vi "核查数据和日志信息出发送队列 (子VI).vi"() -> (0 "错误输出":errorcluster)   [LabVIEW 2016, in "数据传输系统.lvlib"]
uses:
  <vilib>/Utility/config.llb/NI_LVConfig.lvlib
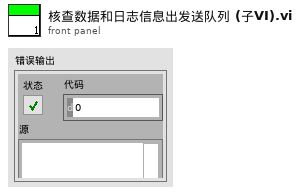
[diagram p1: front panel]
types:
  T1 = enum16{"质控数据", "操作日志", "仪器参数", "系统状态", "运行模式", "测量周期", "超标留样", "报警信息", "环境参数"}
  T2 = enum16{"空白测试", "跨度核查", "标样核查", "加标回收", "平行样", "集成干预"}
  T3 = typedef "NI_LVConfig.lvlib/Config Data RefNum.ctl" = refnum<k1>
  T4 = cluster{"PH":string[][], "CODCr":string[][], "氨氮":string[][], "CODMn":string[][], "总氮":string[][], "总磷":string[][], "电导率":string[][], "水温":string[][], "DO":string[][], "浊度":string[][], "叶绿素":string[][], "藻密度":string[][], "铜":string[][], "盐度":string[][], "水位":string[][], "流速":string[][], "瞬时流量":string[][], "累积流量":string[][]}
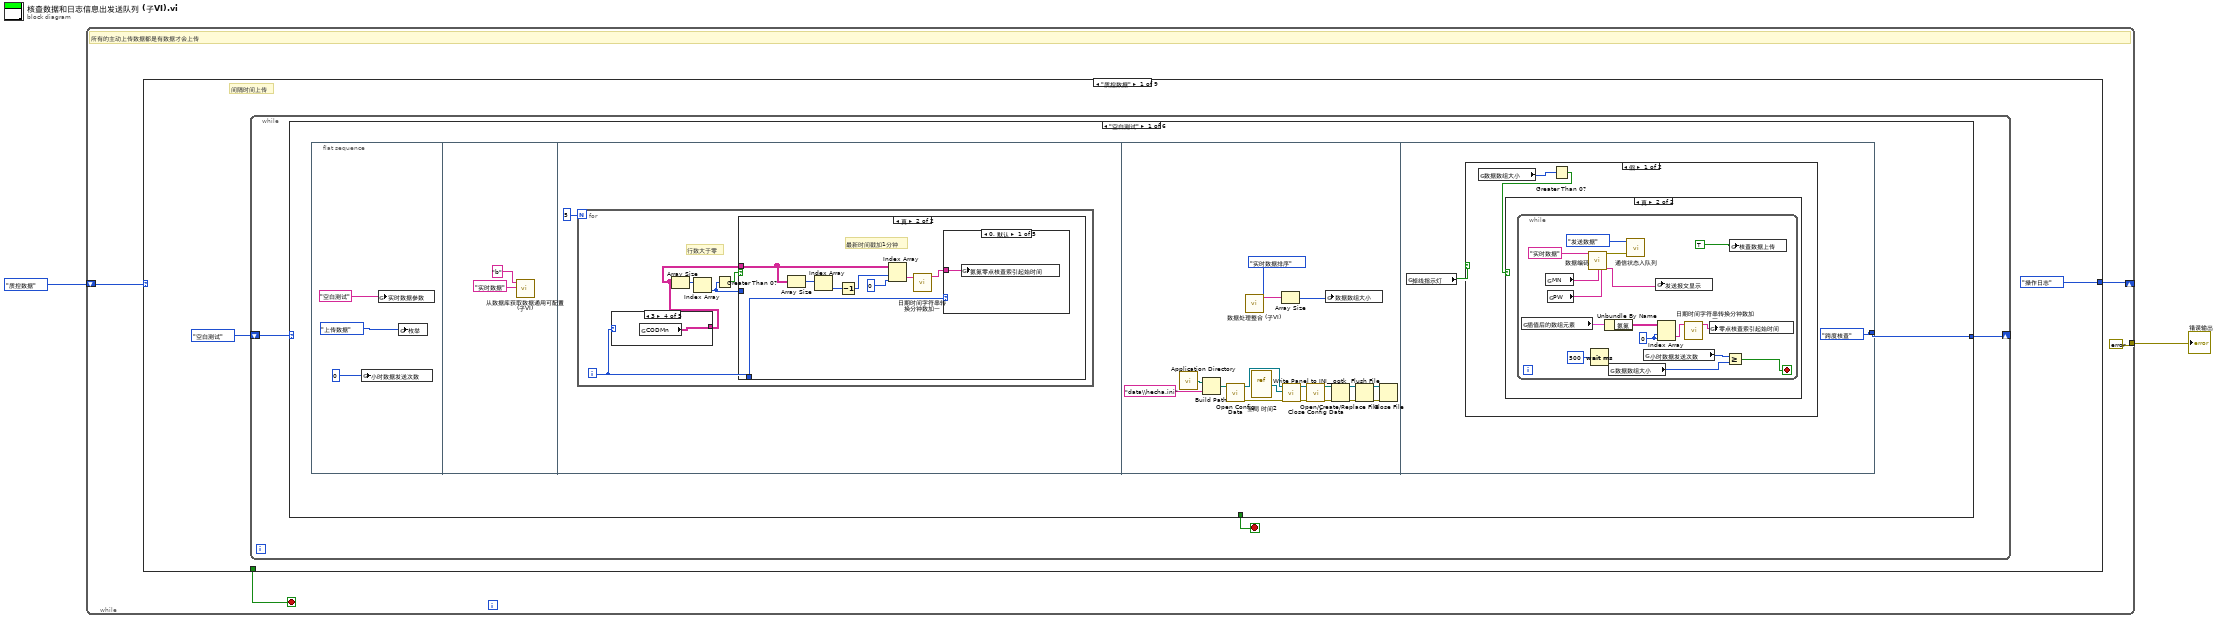
[diagram p0: block diagram]
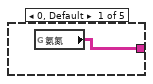
[diagram p2: hidden frame]
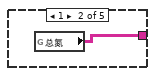
[diagram p3: hidden frame]
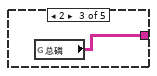
[diagram p4: hidden frame]
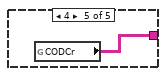
[diagram p5: hidden frame]
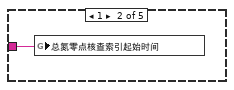
[diagram p7: hidden frame]
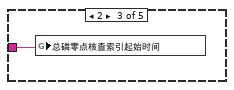
[diagram p8: hidden frame]
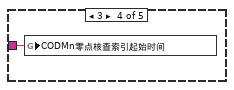
[diagram p9: hidden frame]
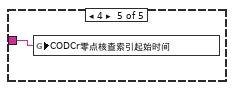
[diagram p10: hidden frame]
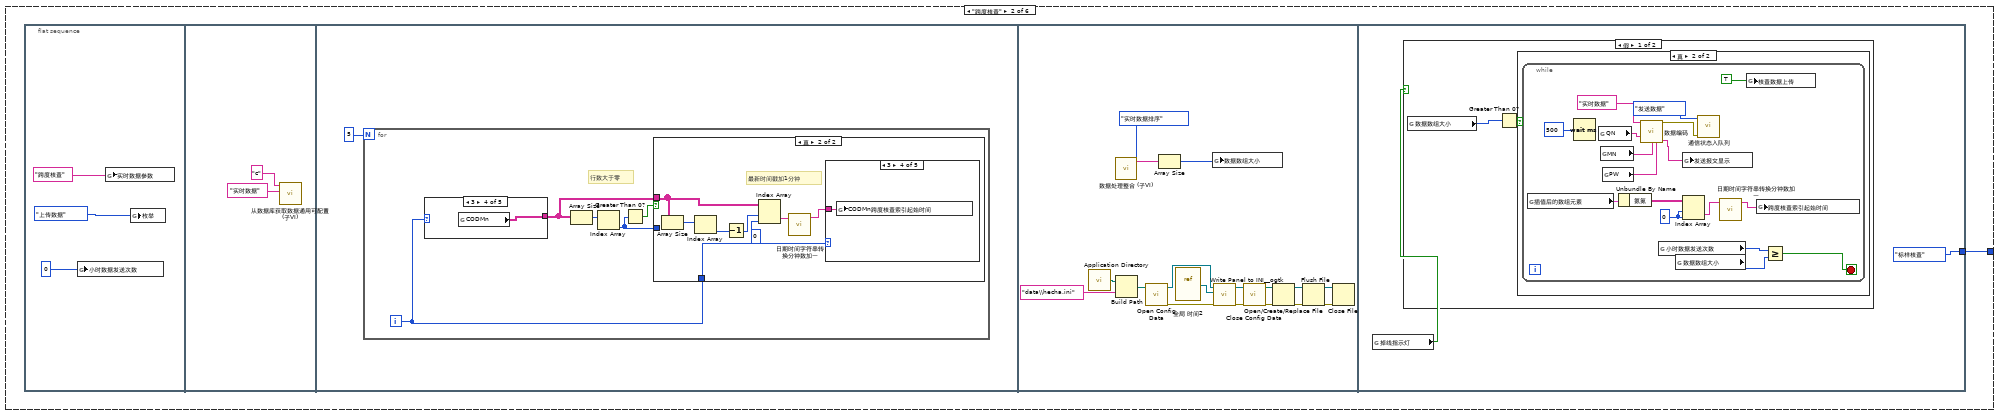
[diagram p13: hidden frame]
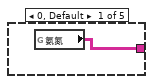
[diagram p14: hidden frame]
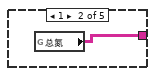
[diagram p15: hidden frame]
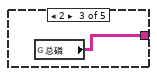
[diagram p16: hidden frame]
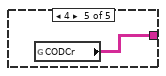
[diagram p17: hidden frame]
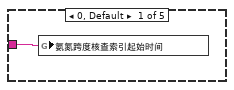
[diagram p19: hidden frame]
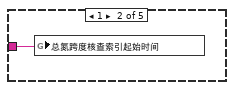
[diagram p20: hidden frame]
diagram:
  n1 = while "While循环" {
    shift-right: [w5] -> _
    shift-left: T1."质控数据" -> [w6]
    tunnel: [errorcluster {"status"=FALSE, "code"=0, "source"=""} ("错误输出")] -> w1
    stop <- w4 stop-if-true
    # "所有的主动上传数据都是有数据才会上传"
    n2 = case shown="\"质控数据\"" w6 {
      tunnel: [T1."操作日志" T1."仪器参数" T1."系统状态" T1."运行模式" T1."测量周期" T1."超标留样" T1."报警信息" T1."环境参数" T1."环境参数"] -> w5
      tunnel: [_ _ _ _ _ _ _ _ TRUE] -> w4
      frame "质控数据" {
        # "间隔时间上传"
        n3 = while {
          shift-right: [w9] -> _
          shift-left: T2."空白测试" -> [w10]
          stop <- w11 stop-if-true
          n4 = case shown="\"空白测试\"" w10 {
            tunnel: [_ _ _ _ _ TRUE] -> w11
            tunnel: [w12 w79 w147 w177 w209 w272] -> w9
            frame "空白测试" {
              n5 = flat-sequence {
                tunnel: [T2."跨度核查"] -> w12
                frame #0 {
                  n6 = global write "全局 小时数据发送次数.vi" "小时数据发送次数"(0 ("小时数据发送次数")) -> ()
                  n7 = global write "全局 实时数据参数.vi" "实时数据参数"("空白测试") -> ()
                  n8 = global write "全局1.vi" "枚举"(enum16{"返回请求应答", "上传数据", "返回执行结果"}."上传数据" ("枚举")) -> ()
                }
                frame #1 {
                  n9 = call "从数据库获取数据通用可配置(子VI).vi"("table输入"="实时数据" ("新元素/子数组"), "列队名（唯一）"="b") -> ()  [unwired: 8 in, 2 out]
                }
                frame #2 {
                  n10 = for {
                    N: 5 -> [_]
                    i -> [w20]
                    # "行数大于零"
                    n11 = case shown="3" w20 {
                      tunnel: [w24 w25 w26 w27 w28] -> w19
                      frame 0, Default {
                        n12 = global read "全局 所有参数.vi" "氨氮"() -> (w24:string[][])
                      }
                      frame 1 {
                        n13 = global read "全局 所有参数.vi" "总氮"() -> (w25:string[][])
                      }
                      frame 2 {
                        n14 = global read "全局 所有参数.vi" "总磷"() -> (w26:string[][])
                      }
                      frame 3 {
                        n15 = global read "全局 所有参数.vi" "CODMn"() -> (w27:string[][])
                      }
                      frame 4 {
                        n16 = global read "全局 所有参数.vi" "CODCr"() -> (w28:string[][])
                      }
                    }
                    n17 = Array Size(array=w19) -> (size(s)=w22:i32[])
                    n18 = Index Array(array=w22) -> (element=w21:i32)  [unwired: 1 in]
                    n19 = Greater Than 0?(x=w21) -> (x > 0?=w23:bool)
                    n20 = case shown="真" w23 {
                      tunnel: w20 -> [_ w36]
                      tunnel: w21 -> [_ _]
                      tunnel: w19 -> [_ w31]
                      frame False {
                      }
                      frame True {
                        # "最新时间戳加1分钟"
                        n21 = Array Size(array=w31) -> (size(s)=w33:i32[])
                        n22 = Index Array(array=w33) -> (element=w32:i32)  [unwired: 1 in]
                        n23 = Decrement(x=w32) -> (x-1=w30:i32)
                        n24 = Index Array(array=w31, index (row)=w30, index (col)=0 ("禁用的索引 (列)")) -> (element=w35:string)
                        n25 = call "日期时间字符串转换分钟数加一.vi"("data[0]"=w35) -> ("日期/时间字符串"=w34:string)  [unwired: 10 in]
                        n26 = case shown="0, 默认" w36 {
                          tunnel: w34 -> [w37 w38 w39 w40 w41]
                          frame 0, Default {
                            n27 = global write "全局 时间2.vi" "氨氮零点核查索引起始时间"(w37) -> ()
                          }
                          frame 1 {
                            n28 = global write "全局 时间2.vi" "总氮零点核查索引起始时间"(w38) -> ()
                          }
                          frame 2 {
                            n29 = global write "全局 时间2.vi" "总磷零点核查索引起始时间"(w39) -> ()
                          }
                          frame 3 {
                            n30 = global write "全局 时间2.vi" "CODMn零点核查索引起始时间"(w40) -> ()
                          }
                          frame 4 {
                            n31 = global write "全局 时间2.vi" "CODCr零点核查索引起始时间"(w41) -> ()
                          }
                        }
                      }
                    }
                  }
                }
                frame #3 {
                  n32 = call <vilib>:"Application Directory.vi"() -> ("Application Directory"=w55:path)
                  n33 = Build Path(base path=w55, name or relative path="data\\hecha.ini" ("名称或相对路径")) -> (appended path=w53:path)
                  n34 = call <vilib>:"Open Config Data.vi"("configuration file path"=w53) -> ("error out"=w49:errorcluster, "refnum"=w52:T3)  [unwired: 8 in, 1 out]
                  n35 = call "数据处理整合 (子VI).vi"("枚举"=enum16{"实时数据排序", "小时数据排序"}."实时数据排序") -> ("已排序的数组"=w58:string[])  [unwired: 10 in]
                  n36 = vi-ref "全局 时间2.vi"() -> (w51:refnum<vi>)
                  n37 = Array Size(array=w58) -> (size(s)=w57:i32)
                  n38 = call <userlib>:"Write Panel to INI__ogtk.vi"("error in (no error)"=w49, "VI ref"=w51, "refnum"=w52) -> ("error out"=w48:errorcluster, "refnum out"=w50:T3)  [unwired: 7 in]
                  n39 = call <vilib>:"Close Config Data.vi"("error in (no error)"=w48, "refnum"=w50) -> ("error out"=w43:errorcluster, "file path"=w42:path)  [unwired: 8 in]
                  n40 = global write "全局 数据数组大小.vi" "数据数组大小"(w57) -> ()
                  n41 = Open/Create/Replace File(file path (use dialog)=w42, error in=w43) -> (refnum out=w46:refnum<file>, error out=w47:errorcluster)  [unwired: 4 in, 1 out]
                  n42 = Flush File(refnum=w46, error in=w47) -> (refnum out=w45:refnum<file>, error out=w44:errorcluster)
                  n43 = Close File(refnum=w45, error in=w44) -> ()  [unwired: 2 out]
                }
                frame #4 {
                  n44 = global read "全局 数据发送重叠.vi" "掉线指示灯"() -> (w60:bool)
                  n45 = case shown="假" w60 {
                    frame False {
                      n46 = global read "全局 数据数组大小.vi" "数据数组大小"() -> (w62:i32)
                      n47 = Greater Than 0?(x=w62) -> (x > 0?=w61:bool)
                      n48 = case shown="真" w61 {
                        frame False {
                        }
                        frame True {
                          n49 = while {
                            stop <- w64 stop-if-true
                            w73 = 0 ("禁用的索引 (列)")
                            n50 = global read "插值后的新数组.vi" "插值后的数组元素"() -> (w77:T4)
                            n51 = global read "断电保存全局.vi" "MN"() -> (w70:string)
                            n52 = global read "断电保存全局.vi" "PW"() -> (w69:string)
                            n53 = call "数据编码.vi"("table输入"="实时数据" ("新元素/子数组"), "MN"=w70, "PW"=w69) -> ("错误常量"=w68:errorcluster, "通讯包字符串"=w72:string)  [unwired: 11 in]
                            n54 = Wait (ms)(milliseconds to wait=u32 500 ("等待时间（毫秒）")) -> ()  [unwired: 1 out]
                            n55 = Unbundle By Name(w77) -> ("氨氮"=w76:string[][])
                            n56 = global read "全局 数据数组大小.vi" "数据数组大小"() -> (w67:i32)
                            n57 = call "通信状态入队列.vi"("错误输入（无错误）"=w68, "枚举"=enum16{"打开连接", "发送数据", "读取数据", "数据处理", "关闭连接"}."发送数据") -> ()  [unwired: 9 in, 1 out]
                            n58 = global read "全局 小时数据发送次数.vi" "小时数据发送次数"() -> (w65:i32)
                            n59 = global write "全局1.vi" "发送报文显示"(w72) -> ()
                            n60 = Index Array(array=w76, index (row)=w73, index (col)=w73) -> (element=w75:string)
                            n61 = call "日期时间字符串转换分钟数加一.vi"("data[0]"=w75) -> ("日期/时间字符串"=w74:string)  [unwired: 10 in]
                            n62 = global write "全局 时间2.vi" "零点核查索引起始时间"(w74) -> ()
                            n63 = Greater Or Equal?(x=w65, y=w67) -> (x >= y?=w64:bool)
                            n64 = global write "全局1.vi" "核查数据上传"(TRUE ("数据上传")) -> ()
                          }
                        }
                      }
                    }
                    frame True {
                    }
                  }
                }
              }
            }
            frame "跨度核查" {
              n65 = flat-sequence {
                tunnel: [T2."标样核查"] -> w79
                frame #0 {
                  n66 = global write "全局 小时数据发送次数.vi" "小时数据发送次数"(0 ("小时数据发送次数")) -> ()
                  n67 = global write "全局 实时数据参数.vi" "实时数据参数"("跨度核查") -> ()
                  n68 = global write "全局1.vi" "枚举"(enum16{"返回请求应答", "上传数据", "返回执行结果"}."上传数据" ("枚举")) -> ()
                }
                frame #1 {
                  n69 = call "从数据库获取数据通用可配置(子VI).vi"("table输入"="实时数据" ("新元素/子数组"), "列队名（唯一）"="c") -> ()  [unwired: 8 in, 2 out]
                }
                frame #2 {
                  n70 = for {
                    N: 5 -> [_]
                    i -> [w86]
                    # "行数大于零"
                    n71 = case shown="3" w86 {
                      tunnel: [w91 w92 w93 w94 w95] -> w87
                      frame 0, Default {
                        n72 = global read "全局 所有参数.vi" "氨氮"() -> (w91:string[][])
                      }
                      frame 1 {
                        n73 = global read "全局 所有参数.vi" "总氮"() -> (w92:string[][])
                      }
                      frame 2 {
                        n74 = global read "全局 所有参数.vi" "总磷"() -> (w93:string[][])
                      }
                      frame 3 {
                        n75 = global read "全局 所有参数.vi" "CODMn"() -> (w94:string[][])
                      }
                      frame 4 {
                        n76 = global read "全局 所有参数.vi" "CODCr"() -> (w95:string[][])
                      }
                    }
                    n77 = Array Size(array=w87) -> (size(s)=w89:i32[])
                    n78 = Index Array(array=w89) -> (element=w88:i32)  [unwired: 1 in]
                    n79 = Greater Than 0?(x=w88) -> (x > 0?=w90:bool)
                    n80 = case shown="真" w90 {
                      tunnel: w86 -> [_ w103]
                      tunnel: w88 -> [_ _]
                      tunnel: w87 -> [_ w97]
                      frame False {
                      }
                      frame True {
                        # "最新时间戳加1分钟"
                        n81 = Array Size(array=w97) -> (size(s)=w100:i32[])
                        n82 = Index Array(array=w100) -> (element=w99:i32)  [unwired: 1 in]
                        n83 = Decrement(x=w99) -> (x-1=w98:i32)
                        n84 = Index Array(array=w97, index (row)=w98, index (col)=0 ("禁用的索引 (列)")) -> (element=w102:string)
                        n85 = call "日期时间字符串转换分钟数加一.vi"("data[0]"=w102) -> ("日期/时间字符串"=w101:string)  [unwired: 10 in]
                        n86 = case shown="3" w103 {
                          tunnel: w101 -> [w104 w105 w106 w107 w108]
                          frame 0, Default {
                            n87 = global write "全局 时间2.vi" "氨氮跨度核查索引起始时间"(w104) -> ()
                          }
                          frame 1 {
                            n88 = global write "全局 时间2.vi" "总氮跨度核查索引起始时间"(w105) -> ()
                          }
                          frame 2 {
                            n89 = global write "全局 时间2.vi" "总磷跨度核查索引起始时间"(w106) -> ()
                          }
                          frame 3 {
                            n90 = global write "全局 时间2.vi" "CODMn跨度核查索引起始时间"(w107) -> ()
                          }
                          frame 4 {
                            n91 = global write "全局 时间2.vi" "CODCr跨度核查索引起始时间"(w108) -> ()
                          }
                        }
                      }
                    }
                  }
                }
                frame #3 {
                  n92 = call <vilib>:"Application Directory.vi"() -> ("Application Directory"=w122:path)
                  n93 = call "数据处理整合 (子VI).vi"("枚举"=enum16{"实时数据排序", "小时数据排序"}."实时数据排序") -> ("已排序的数组"=w125:string[])  [unwired: 10 in]
                  n94 = Build Path(base path=w122, name or relative path="data\\hecha.ini" ("名称或相对路径")) -> (appended path=w120:path)
                  n95 = call <vilib>:"Open Config Data.vi"("configuration file path"=w120) -> ("error out"=w116:errorcluster, "refnum"=w119:T3)  [unwired: 8 in, 1 out]
                  n96 = Array Size(array=w125) -> (size(s)=w124:i32)
                  n97 = vi-ref "全局 时间2.vi"() -> (w118:refnum<vi>)
                  n98 = global write "全局 数据数组大小.vi" "数据数组大小"(w124) -> ()
                  n99 = call <userlib>:"Write Panel to INI__ogtk.vi"("error in (no error)"=w116, "VI ref"=w118, "refnum"=w119) -> ("error out"=w115:errorcluster, "refnum out"=w117:T3)  [unwired: 7 in]
                  n100 = call <vilib>:"Close Config Data.vi"("error in (no error)"=w115, "refnum"=w117) -> ("error out"=w110:errorcluster, "file path"=w109:path)  [unwired: 8 in]
                  n101 = Open/Create/Replace File(file path (use dialog)=w109, error in=w110) -> (refnum out=w113:refnum<file>, error out=w114:errorcluster)  [unwired: 4 in, 1 out]
                  n102 = Flush File(refnum=w113, error in=w114) -> (refnum out=w112:refnum<file>, error out=w111:errorcluster)
                  n103 = Close File(refnum=w112, error in=w111) -> ()  [unwired: 2 out]
                }
                frame #4 {
                  n104 = global read "全局 数据发送重叠.vi" "掉线指示灯"() -> (w127:bool)
                  n105 = case shown="假" w127 {
                    frame False {
                      n106 = global read "全局 数据数组大小.vi" "数据数组大小"() -> (w129:i32)
                      n107 = Greater Than 0?(x=w129) -> (x > 0?=w128:bool)
                      n108 = case shown="真" w128 {
                        frame False {
                        }
                        frame True {
                          n109 = while {
                            stop <- w131 stop-if-true
                            w141 = 0 ("禁用的索引 (列)")
                            n110 = global read "插值后的新数组.vi" "插值后的数组元素"() -> (w145:T4)
                            n111 = Wait (ms)(milliseconds to wait=u32 500 ("等待时间（毫秒）")) -> ()  [unwired: 1 out]
                            n112 = global read "全局1.vi" "QN"() -> (w140:string)
                            n113 = global read "断电保存全局.vi" "MN"() -> (w138:string)
                            n114 = global read "断电保存全局.vi" "PW"() -> (w137:string)
                            n115 = Unbundle By Name(w145) -> ("氨氮"=w144:string[][])
                            n116 = call "数据编码.vi"("table输入"="实时数据" ("新元素/子数组"), "QN"=w140, "MN"=w138, "PW"=w137) -> ("错误常量"=w135:errorcluster, "通讯包字符串"=w136:string)  [unwired: 10 in]
                            n117 = global read "全局 小时数据发送次数.vi" "小时数据发送次数"() -> (w132:i32)
                            n118 = global read "全局 数据数组大小.vi" "数据数组大小"() -> (w133:i32)
                            n119 = Index Array(array=w144, index (row)=w141, index (col)=w141) -> (element=w143:string)
                            n120 = global write "全局1.vi" "发送报文显示"(w136) -> ()
                            n121 = call "通信状态入队列.vi"("错误输入（无错误）"=w135, "枚举"=enum16{"打开连接", "发送数据", "读取数据", "数据处理", "关闭连接"}."发送数据") -> ()  [unwired: 9 in, 1 out]
                            n122 = call "日期时间字符串转换分钟数加一.vi"("data[0]"=w143) -> ("日期/时间字符串"=w142:string)  [unwired: 10 in]
                            n123 = global write "全局1.vi" "核查数据上传"(TRUE ("数据上传")) -> ()
                            n124 = global write "全局 时间2.vi" "跨度核查索引起始时间"(w142) -> ()
                            n125 = Greater Or Equal?(x=w132, y=w133) -> (x >= y?=w131:bool)
                          }
                        }
                      }
                    }
                    frame True {
                    }
                  }
                }
              }
            }
            frame "标样核查" {
              n126 = flat-sequence {
                tunnel: [T2."加标回收"] -> w147
                frame #0 {
                  n127 = global write "全局 小时数据发送次数.vi" "小时数据发送次数"(0 ("小时数据发送次数")) -> ()
                  n128 = global write "全局 实时数据参数.vi" "实时数据参数"("核查数据") -> ()
                  n129 = global write "全局1.vi" "枚举"(enum16{"返回请求应答", "上传数据", "返回执行结果"}."上传数据" ("枚举")) -> ()
                }
                frame #1 {
                  n130 = call "从数据库获取数据通用可配置(子VI).vi"("table输入"="实时数据" ("新元素/子数组"), "列队名（唯一）"="n") -> ()  [unwired: 8 in, 2 out]
                }
                frame #2 {
                  n131 = call "数据处理整合 (子VI).vi"("枚举"=enum16{"实时数据排序", "小时数据排序"}."实时数据排序") -> ("已排序的数组"=w155:string[])  [unwired: 10 in]
                  n132 = Array Size(array=w155) -> (size(s)=w154:i32)
                  n133 = global write "全局 数据数组大小.vi" "数据数组大小"(w154) -> ()
                }
                frame #3 {
                  n134 = global read "全局 数据发送重叠.vi" "掉线指示灯"() -> (w157:bool)
                  n135 = case shown="假" w157 {
                    frame False {
                      n136 = global read "全局 数据数组大小.vi" "数据数组大小"() -> (w159:i32)
                      n137 = Greater Than 0?(x=w159) -> (x > 0?=w158:bool)
                      n138 = case shown="真" w158 {
                        frame False {
                        }
                        frame True {
                          n139 = while {
                            stop <- w162 stop-if-true
                            w171 = 0 ("禁用的索引 (列)")
                            n140 = global read "插值后的新数组.vi" "插值后的数组元素"() -> (w175:T4)
                            n141 = global read "全局1.vi" "QN"() -> (w170:string)
                            n142 = global read "断电保存全局.vi" "MN"() -> (w167:string)
                            n143 = global read "断电保存全局.vi" "PW"() -> (w166:string)
                            n144 = Unbundle By Name(w175) -> ("氨氮"=w174:string[][])
                            n145 = call "数据编码.vi"("table输入"="实时数据" ("新元素/子数组"), "QN"=w170, "MN"=w167, "PW"=w166) -> ("错误常量"=w165:errorcluster, "通讯包字符串"=w169:string)  [unwired: 10 in]
                            n146 = global read "全局 小时数据发送次数.vi" "小时数据发送次数"() -> (w163:i32)
                            n147 = global write "全局1.vi" "发送报文显示"(w169) -> ()
                            n148 = global read "全局 数据数组大小.vi" "数据数组大小"() -> (w164:i32)
                            n149 = Index Array(array=w174, index (row)=w171, index (col)=w171) -> (element=w173:string)
                            n150 = call "通信状态入队列.vi"("错误输入（无错误）"=w165, "枚举"=enum16{"打开连接", "发送数据", "读取数据", "数据处理", "关闭连接"}."发送数据") -> ()  [unwired: 9 in, 1 out]
                            n151 = call "日期时间字符串转换分钟数加一.vi"("data[0]"=w173) -> ("日期/时间字符串"=w172:string)  [unwired: 10 in]
                            n152 = global write "全局1.vi" "核查数据上传"(TRUE ("数据上传")) -> ()
                            n153 = global write "全局 时间2.vi" "标样核查索引起始时间"(w172) -> ()
                            n154 = Greater Or Equal?(x=w163, y=w164) -> (x >= y?=w162:bool)
                            n155 = Wait (ms)(milliseconds to wait=u32 500 ("等待时间（毫秒）")) -> ()  [unwired: 1 out]
                          }
                        }
                      }
                    }
                    frame True {
                    }
                  }
                }
              }
            }
            frame "加标回收" {
              n156 = flat-sequence {
                tunnel: [T2."平行样"] -> w177
                frame #0 {
                  n157 = global write "全局 小时数据发送次数.vi" "小时数据发送次数"(0 ("小时数据发送次数")) -> ()
                  n158 = global write "全局 实时数据参数.vi" "实时数据参数"("加标回收测试") -> ()
                  n159 = global write "全局1.vi" "枚举"(enum16{"返回请求应答", "上传数据", "返回执行结果"}."上传数据" ("枚举")) -> ()
                }
                frame #1 {
                  n160 = call "从数据库获取数据通用可配置(子VI).vi"("table输入"="加标回收" ("新元素/子数组"), "列队名（唯一）"="d") -> ()  [unwired: 8 in, 2 out]
                }
                frame #2 {
                  n161 = call "加标回收数据处理整合 (子VI).vi"("枚举"=enum16{"实时数据排序", "小时数据排序"}."实时数据排序") -> ("已排序的数组"=w184:string[])  [unwired: 10 in]
                  n162 = Array Size(array=w184) -> (size(s)=w185:i32)
                  n163 = global write "全局 数据数组大小.vi" "数据数组大小"(w185) -> ()
                }
                frame #3 {
                  n164 = global read "全局 数据发送重叠.vi" "掉线指示灯"() -> (w187:bool)
                  n165 = case shown="假" w187 {
                    frame False {
                      n166 = global read "全局 数据数组大小.vi" "数据数组大小"() -> (w189:i32)
                      n167 = Greater Than 0?(x=w189) -> (x > 0?=w188:bool)
                      n168 = case shown="真" w188 {
                        frame False {
                        }
                        frame True {
                          n169 = while {
                            stop <- w192 stop-if-true
                            n170 = global read "全局 数据数组大小.vi" "数据数组大小"() -> (w204:i32)
                            n171 = global read "插值后的新数组.vi" "插值后的数组元素"() -> (w207:T4)
                            n172 = global read "全局1.vi" "QN"() -> (w200:string)
                            n173 = global read "断电保存全局.vi" "MN"() -> (w197:string)
                            n174 = global read "断电保存全局.vi" "PW"() -> (w196:string)
                            n175 = Decrement(x=w204) -> (x-1=w203:i32)
                            n176 = call "数据编码.vi"("table输入"="实时数据" ("新元素/子数组"), "QN"=w200, "MN"=w197, "PW"=w196) -> ("错误常量"=w195:errorcluster, "通讯包字符串"=w199:string)  [unwired: 10 in]
                            n177 = Unbundle By Name(w207) -> ("氨氮"=w206:string[][])
                            n178 = global write "全局1.vi" "发送报文显示"(w199) -> ()
                            n179 = call "通信状态入队列.vi"("错误输入（无错误）"=w195, "枚举"=enum16{"打开连接", "发送数据", "读取数据", "数据处理", "关闭连接"}."发送数据") -> ()  [unwired: 9 in, 1 out]
                            n180 = global read "全局 小时数据发送次数.vi" "小时数据发送次数"() -> (w193:i32)
                            n181 = Index Array(array=w206, index (row)=w203, index (col)=0 ("禁用的索引 (列)")) -> (element=w202:string)
                            n182 = global read "全局 数据数组大小.vi" "数据数组大小"() -> (w194:i32)
                            n183 = call "日期时间字符串转换分钟数加一.vi"("data[0]"=w202) -> ("日期/时间字符串"=w201:string)  [unwired: 10 in]
                            n184 = global write "全局 时间2.vi" "加标回收索引起始时间"(w201) -> ()
                            n185 = global write "全局1.vi" "核查数据上传"(TRUE ("数据上传")) -> ()
                            n186 = Greater Or Equal?(x=w193, y=w194) -> (x >= y?=w192:bool)
                            n187 = Wait (ms)(milliseconds to wait=u32 500 ("等待时间（毫秒）")) -> ()  [unwired: 1 out]
                          }
                        }
                      }
                    }
                    frame True {
                    }
                  }
                }
              }
            }
            frame "平行样" {
              n188 = flat-sequence {
                tunnel: [T2."集成干预"] -> w209
                frame #0 {
                  n189 = global write "全局 小时数据发送次数.vi" "小时数据发送次数"(0 ("小时数据发送次数")) -> ()
                  n190 = global write "全局 实时数据参数.vi" "实时数据参数"("平行样测试") -> ()
                  n191 = global write "全局1.vi" "枚举"(enum16{"返回请求应答", "上传数据", "返回执行结果"}."上传数据" ("枚举")) -> ()
                }
                frame #1 {
                  n192 = call "从数据库获取数据通用可配置(子VI).vi"("table输入"="平行样测试" ("新元素/子数组"), "列队名（唯一）"="e") -> ()  [unwired: 8 in, 2 out]
                }
                frame #2 {
                  n193 = for {
                    N: 5 -> [_]
                    i -> [w216]
                    # "行数大于零"
                    n194 = case shown="3" w216 {
                      tunnel: [w221 w222 w223 w224 w225] -> w217
                      frame 0, Default {
                        n195 = global read "全局 所有参数.vi" "氨氮"() -> (w221:string[][])
                      }
                      frame 1 {
                        n196 = global read "全局 所有参数.vi" "总氮"() -> (w222:string[][])
                      }
                      frame 2 {
                        n197 = global read "全局 所有参数.vi" "总磷"() -> (w223:string[][])
                      }
                      frame 3 {
                        n198 = global read "全局 所有参数.vi" "CODMn"() -> (w224:string[][])
                      }
                      frame 4 {
                        n199 = global read "全局 所有参数.vi" "CODCr"() -> (w225:string[][])
                      }
                    }
                    n200 = Array Size(array=w217) -> (size(s)=w219:i32[])
                    n201 = Index Array(array=w219) -> (element=w218:i32)  [unwired: 1 in]
                    n202 = Greater Than 0?(x=w218) -> (x > 0?=w220:bool)
                    n203 = case shown="真" w220 {
                      tunnel: w216 -> [_ w233]
                      tunnel: w218 -> [_ _]
                      tunnel: w217 -> [_ w228]
                      frame False {
                      }
                      frame True {
                        # "最新时间戳加1分钟"
                        n204 = Array Size(array=w228) -> (size(s)=w230:i32[])
                        n205 = Index Array(array=w230) -> (element=w229:i32)  [unwired: 1 in]
                        n206 = Decrement(x=w229) -> (x-1=w227:i32)
                        n207 = Index Array(array=w228, index (row)=w227, index (col)=0 ("禁用的索引 (列)")) -> (element=w232:string)
                        n208 = call "日期时间字符串转换分钟数加一.vi"("data[0]"=w232) -> ("日期/时间字符串"=w231:string)  [unwired: 10 in]
                        n209 = case shown="0, 默认" w233 {
                          tunnel: w231 -> [w234 w235 w236 w237 w238]
                          frame 0, Default {
                            n210 = global write "全局 时间2.vi" "氨氮平行样索引起始时间"(w234) -> ()
                          }
                          frame 1 {
                            n211 = global write "全局 时间2.vi" "总氮平行样索引起始时间"(w235) -> ()
                          }
                          frame 2 {
                            n212 = global write "全局 时间2.vi" "总磷平行样索引起始时间"(w236) -> ()
                          }
                          frame 3 {
                            n213 = global write "全局 时间2.vi" "CODMn平行样索引起始时间"(w237) -> ()
                          }
                          frame 4 {
                            n214 = global write "全局 时间2.vi" "CODCr平行样索引起始时间"(w238) -> ()
                          }
                        }
                      }
                    }
                  }
                }
                frame #3 {
                  n215 = call "数据处理整合 (子VI).vi"("枚举"=enum16{"实时数据排序", "小时数据排序"}."实时数据排序") -> ("已排序的数组"=w255:string[])  [unwired: 10 in]
                  n216 = Array Size(array=w255) -> (size(s)=w254:i32)
                  n217 = call <vilib>:"Application Directory.vi"() -> ("Application Directory"=w252:path)
                  n218 = Build Path(base path=w252, name or relative path="data\\hecha.ini" ("名称或相对路径")) -> (appended path=w250:path)
                  n219 = global write "全局 数据数组大小.vi" "数据数组大小"(w254) -> ()
                  n220 = call <vilib>:"Open Config Data.vi"("configuration file path"=w250) -> ("error out"=w246:errorcluster, "refnum"=w249:T3)  [unwired: 8 in, 1 out]
                  n221 = vi-ref "全局 时间2.vi"() -> (w248:refnum<vi>)
                  n222 = call <userlib>:"Write Panel to INI__ogtk.vi"("error in (no error)"=w246, "VI ref"=w248, "refnum"=w249) -> ("error out"=w245:errorcluster, "refnum out"=w247:T3)  [unwired: 7 in]
                  n223 = call <vilib>:"Close Config Data.vi"("error in (no error)"=w245, "refnum"=w247) -> ("error out"=w240:errorcluster, "file path"=w239:path)  [unwired: 8 in]
                  n224 = Open/Create/Replace File(file path (use dialog)=w239, error in=w240) -> (refnum out=w243:refnum<file>, error out=w244:errorcluster)  [unwired: 4 in, 1 out]
                  n225 = Flush File(refnum=w243, error in=w244) -> (refnum out=w242:refnum<file>, error out=w241:errorcluster)
                  n226 = Close File(refnum=w242, error in=w241) -> ()  [unwired: 2 out]
                }
                frame #4 {
                  n227 = global read "全局 数据发送重叠.vi" "掉线指示灯"() -> (w256:bool)
                  n228 = case shown="假" w256 {
                    frame False {
                      n229 = global read "全局 数据数组大小.vi" "数据数组大小"() -> (w259:i32)
                      n230 = Greater Than 0?(x=w259) -> (x > 0?=w258:bool)
                      n231 = case shown="真" w258 {
                        frame False {
                        }
                        frame True {
                          n232 = while {
                            stop <- w262 stop-if-true
                            n233 = global read "全局1.vi" "QN"() -> (w270:string)
                            n234 = global read "断电保存全局.vi" "MN"() -> (w267:string)
                            n235 = global read "断电保存全局.vi" "PW"() -> (w266:string)
                            n236 = global read "全局 小时数据发送次数.vi" "小时数据发送次数"() -> (w263:i32)
                            n237 = global read "全局 数据数组大小.vi" "数据数组大小"() -> (w264:i32)
                            n238 = call "数据编码.vi"("table输入"="实时数据" ("新元素/子数组"), "QN"=w270, "MN"=w267, "PW"=w266) -> ("错误常量"=w265:errorcluster, "通讯包字符串"=w269:string)  [unwired: 10 in]
                            n239 = global write "全局1.vi" "核查数据上传"(TRUE ("数据上传")) -> ()
                            n240 = global write "全局1.vi" "发送报文显示"(w269) -> ()
                            n241 = call "通信状态入队列.vi"("错误输入（无错误）"=w265, "枚举"=enum16{"打开连接", "发送数据", "读取数据", "数据处理", "关闭连接"}."发送数据") -> ()  [unwired: 9 in, 1 out]
                            n242 = Greater Or Equal?(x=w263, y=w264) -> (x >= y?=w262:bool)
                            n243 = Wait (ms)(milliseconds to wait=u32 500 ("等待时间（毫秒）")) -> ()  [unwired: 1 out]
                          }
                        }
                      }
                    }
                    frame True {
                    }
                  }
                }
              }
            }
            frame "集成干预" {
              n244 = flat-sequence {
                tunnel: [T2."集成干预"] -> w272
                frame #0 {
                  n245 = global write "全局 小时数据发送次数.vi" "小时数据发送次数"(0 ("小时数据发送次数")) -> ()
                  n246 = global write "全局 实时数据参数.vi" "实时数据参数"("集成干预测试") -> ()
                  n247 = global write "全局1.vi" "枚举"(enum16{"返回请求应答", "上传数据", "返回执行结果"}."上传数据" ("枚举")) -> ()
                }
                frame #1 {
                  n248 = call "从数据库获取数据通用可配置(子VI).vi"("table输入"="集成干预测试" ("新元素/子数组"), "列队名（唯一）"="f") -> ()  [unwired: 8 in, 2 out]
                }
                frame #2 {
                  n249 = for {
                    N: 12 -> [_]
                    i -> [w280]
                    # "行数大于零"
                    n250 = case shown="10" w280 {
                      tunnel: [w285 w286 w287 w288 w289 w290 w291 w292 w293 w294 w295 w296] -> w281
                      frame 0, Default {
                        n251 = global read "全局 所有参数.vi" "氨氮"() -> (w285:string[][])
                      }
                      frame 1 {
                        n252 = global read "全局 所有参数.vi" "总氮"() -> (w286:string[][])
                      }
                      frame 2 {
                        n253 = global read "全局 所有参数.vi" "总磷"() -> (w287:string[][])
                      }
                      frame 3 {
                        n254 = global read "全局 所有参数.vi" "CODMn"() -> (w288:string[][])
                      }
                      frame 4 {
                        n255 = global read "全局 所有参数.vi" "CODCr"() -> (w289:string[][])
                      }
                      frame 5 {
                        n256 = global read "全局 所有参数.vi" "DO"() -> (w290:string[][])
                      }
                      frame 6 {
                        n257 = global read "全局 所有参数.vi" "PH"() -> (w291:string[][])
                      }
                      frame 7 {
                        n258 = global read "全局 所有参数.vi" "电导率"() -> (w292:string[][])
                      }
                      frame 8 {
                        n259 = global read "全局 所有参数.vi" "水温"() -> (w293:string[][])
                      }
                      frame 9 {
                        n260 = global read "全局 所有参数.vi" "浊度"() -> (w294:string[][])
                      }
                      frame 10 {
                        n261 = global read "全局 所有参数.vi" "叶绿素"() -> (w295:string[][])
                      }
                      frame 11 {
                        n262 = global read "全局 所有参数.vi" "藻密度"() -> (w296:string[][])
                      }
                    }
                    n263 = Array Size(array=w281) -> (size(s)=w283:i32[])
                    n264 = Index Array(array=w283) -> (element=w282:i32)  [unwired: 1 in]
                    n265 = Greater Than 0?(x=w282) -> (x > 0?=w284:bool)
                    n266 = case shown="真" w284 {
                      tunnel: w280 -> [_ w304]
                      tunnel: w282 -> [_ _]
                      tunnel: w281 -> [_ w297]
                      frame False {
                      }
                      frame True {
                        # "最新时间戳加1分钟"
                        n267 = Array Size(array=w297) -> (size(s)=w301:i32[])
                        n268 = Index Array(array=w301) -> (element=w300:i32)  [unwired: 1 in]
                        n269 = Decrement(x=w300) -> (x-1=w299:i32)
                        n270 = Index Array(array=w297, index (row)=w299, index (col)=0 ("禁用的索引 (列)")) -> (element=w303:string)
                        n271 = call "日期时间字符串转换分钟数加一.vi"("data[0]"=w303) -> ("日期/时间字符串"=w302:string)  [unwired: 10 in]
                        n272 = case shown="10" w304 {
                          tunnel: w302 -> [w305 w306 w307 w308 w309 w310 w311 w312 w313 w314 w315 w316]
                          frame 0, Default {
                            n273 = global write "全局 时间2.vi" "氨氮集成干预索引起始时间"(w305) -> ()
                          }
                          frame 1 {
                            n274 = global write "全局 时间2.vi" "总氮集成干预索引起始时间"(w306) -> ()
                          }
                          frame 2 {
                            n275 = global write "全局 时间2.vi" "总磷集成干预索引起始时间"(w307) -> ()
                          }
                          frame 3 {
                            n276 = global write "全局 时间2.vi" "CODMn集成干预索引起始时间"(w308) -> ()
                          }
                          frame 4 {
                            n277 = global write "全局 时间2.vi" "CODCr集成干预索引起始时间"(w309) -> ()
                          }
                          frame 5 {
                            n278 = global write "全局 时间2.vi" "DO集成干预索引起始时间"(w310) -> ()
                          }
                          frame 6 {
                            n279 = global write "全局 时间2.vi" "PH集成干预索引起始时间"(w311) -> ()
                          }
                          frame 7 {
                            n280 = global write "全局 时间2.vi" "比电导率集成干预索引起始时间"(w312) -> ()
                          }
                          frame 8 {
                            n281 = global write "全局 时间2.vi" "水温集成干预索引起始时间"(w313) -> ()
                          }
                          frame 9 {
                            n282 = global write "全局 时间2.vi" "浊度集成干预索引起始时间"(w314) -> ()
                          }
                          frame 10 {
                            n283 = global write "全局 时间2.vi" "叶绿素a集成干预索引起始时间"(w315) -> ()
                          }
                          frame 11 {
                            n284 = global write "全局 时间2.vi" "藻密度集成干预索引起始时间"(w316) -> ()
                          }
                        }
                      }
                    }
                  }
                }
                frame #3 {
                  n285 = call "数据处理整合 (子VI).vi"("枚举"=enum16{"实时数据排序", "小时数据排序"}."实时数据排序") -> ("已排序的数组"=w333:string[])  [unwired: 10 in]
                  n286 = Array Size(array=w333) -> (size(s)=w332:i32)
                  n287 = call <vilib>:"Application Directory.vi"() -> ("Application Directory"=w330:path)
                  n288 = Build Path(base path=w330, name or relative path="data\\hecha.ini" ("名称或相对路径")) -> (appended path=w328:path)
                  n289 = global write "全局 数据数组大小.vi" "数据数组大小"(w332) -> ()
                  n290 = call <vilib>:"Open Config Data.vi"("configuration file path"=w328) -> ("error out"=w324:errorcluster, "refnum"=w327:T3)  [unwired: 8 in, 1 out]
                  n291 = vi-ref "全局 时间2.vi"() -> (w326:refnum<vi>)
                  n292 = call <userlib>:"Write Panel to INI__ogtk.vi"("error in (no error)"=w324, "VI ref"=w326, "refnum"=w327) -> ("error out"=w323:errorcluster, "refnum out"=w325:T3)  [unwired: 7 in]
                  n293 = call <vilib>:"Close Config Data.vi"("error in (no error)"=w323, "refnum"=w325) -> ("error out"=w318:errorcluster, "file path"=w317:path)  [unwired: 8 in]
                  n294 = Open/Create/Replace File(file path (use dialog)=w317, error in=w318) -> (refnum out=w321:refnum<file>, error out=w322:errorcluster)  [unwired: 4 in, 1 out]
                  n295 = Flush File(refnum=w321, error in=w322) -> (refnum out=w320:refnum<file>, error out=w319:errorcluster)
                  n296 = Close File(refnum=w320, error in=w319) -> ()  [unwired: 2 out]
                }
                frame #4 {
                  n297 = global read "全局 数据发送重叠.vi" "掉线指示灯"() -> (w335:bool)
                  n298 = case shown="假" w335 {
                    frame False {
                      n299 = global read "全局 数据数组大小.vi" "数据数组大小"() -> (w337:i32)
                      n300 = Greater Than 0?(x=w337) -> (x > 0?=w336:bool)
                      n301 = case shown="真" w336 {
                        frame False {
                        }
                        frame True {
                          n302 = while {
                            stop <- w340 stop-if-true
                            n303 = global read "全局1.vi" "QN"() -> (w348:string)
                            n304 = global read "断电保存全局.vi" "MN"() -> (w344:string)
                            n305 = global read "断电保存全局.vi" "PW"() -> (w343:string)
                            n306 = global read "全局 数据数组大小.vi" "数据数组大小"() -> (w342:i32)
                            n307 = global read "全局 小时数据发送次数.vi" "小时数据发送次数"() -> (w341:i32)
                            n308 = call "数据编码.vi"("table输入"="实时数据" ("新元素/子数组"), "QN"=w348, "MN"=w344, "PW"=w343) -> ("错误常量"=w345:errorcluster, "通讯包字符串"=w347:string)  [unwired: 10 in]
                            n309 = global write "全局1.vi" "核查数据上传"(TRUE ("数据上传")) -> ()
                            n310 = call "通信状态入队列.vi"("错误输入（无错误）"=w345, "枚举"=enum16{"打开连接", "发送数据", "读取数据", "数据处理", "关闭连接"}."发送数据") -> ()  [unwired: 9 in, 1 out]
                            n311 = global write "全局1.vi" "发送报文显示"(w347) -> ()
                            n312 = Greater Or Equal?(x=w341, y=w342) -> (x >= y?=w340:bool)
                            n313 = Wait (ms)(milliseconds to wait=u32 500 ("等待时间（毫秒）")) -> ()  [unwired: 1 out]
                          }
                        }
                      }
                    }
                    frame True {
                    }
                  }
                }
              }
            }
          }
        }
      }
      frame "操作日志" {
        # "间隔时间上传"
        # "直接1分钟查询 一次,有数据就按数据上传,没数据就不上传,在数据发送那边有做处理"
        n314 = flat-sequence {
          frame #0 {
            # "时间"
            n315 = global write "全局 小时数据发送次数.vi" "小时数据发送次数"(0 ("小时数据发送次数")) -> ()
            n316 = call "日志信息主动发送(子VI).vi"() -> ()  [unwired: 12 in]
            n317 = global write "全局1.vi" "枚举"(enum16{"返回请求应答", "上传数据", "返回执行结果"}."上传数据" ("枚举")) -> ()
          }
          frame #1 {
            n318 = call "获取操作日志 (子VI).vi"("table输入"="操作日志") -> ()  [unwired: 11 in]
          }
          frame #2 {
            n319 = for {
              N: 6 -> [_]
              i -> [w356]
              # "行数大于零"
              n320 = case shown="0, 默认" w356 {
                tunnel: [w360 w361 w362 w363 w364 w365] -> w355
                frame 0, Default {
                  n321 = global read "全局 所有参数.vi" "氨氮"() -> (w360:string[][])
                }
                frame 1 {
                  n322 = global read "全局 所有参数.vi" "总氮"() -> (w361:string[][])
                }
                frame 2 {
                  n323 = global read "全局 所有参数.vi" "总磷"() -> (w362:string[][])
                }
                frame 3 {
                  n324 = global read "全局 所有参数.vi" "CODMn"() -> (w363:string[][])
                }
                frame 4 {
                  n325 = global read "全局 所有参数.vi" "CODCr"() -> (w364:string[][])
                }
                frame 5 {
                  n326 = global read "全局 所有参数.vi" "DO"() -> (w365:string[][])
                }
              }
              n327 = Array Size(array=w355) -> (size(s)=w358:i32[])
              n328 = Index Array(array=w358) -> (element=w357:i32)  [unwired: 1 in]
              n329 = Greater Than 0?(x=w357) -> (x > 0?=w359:bool)
              n330 = case shown="真" w359 {
                tunnel: w356 -> [_ w373]
                tunnel: w357 -> [_ _]
                tunnel: w355 -> [_ w368]
                frame False {
                }
                frame True {
                  # "最新时间戳加1分钟"
                  n331 = Array Size(array=w368) -> (size(s)=w370:i32[])
                  n332 = Index Array(array=w370) -> (element=w369:i32)  [unwired: 1 in]
                  n333 = Decrement(x=w369) -> (x-1=w367:i32)
                  n334 = Index Array(array=w368, index (row)=w367, index (col)=0 ("禁用的索引 (列)")) -> (element=w372:string)
                  n335 = call "日期时间字符串转换分钟数加一.vi"("data[0]"=w372) -> ("日期/时间字符串"=w371:string)  [unwired: 10 in]
                  n336 = case shown="5" w373 {
                    tunnel: w371 -> [w374 w375 w376 w377 w378 w379]
                    frame 0, Default {
                      n337 = global write "全局 时间2.vi" "氨氮仪器日志索引起始时间"(w374) -> ()
                    }
                    frame 1 {
                      n338 = global write "全局 时间2.vi" "总氮仪器日志索引起始时间"(w375) -> ()
                    }
                    frame 2 {
                      n339 = global write "全局 时间2.vi" "总磷仪器日志索引起始时间"(w376) -> ()
                    }
                    frame 3 {
                      n340 = global write "全局 时间2.vi" "CODMn仪器日志索引起始时间"(w377) -> ()
                    }
                    frame 4 {
                      n341 = global write "全局 时间2.vi" "CODCr仪器日志索引起始时间"(w378) -> ()
                    }
                    frame 5 {
                      n342 = global write "全局 时间2.vi" "系统仪器日志索引起始时间"(w379) -> ()
                    }
                  }
                }
              }
            }
          }
          frame #3 {
            n343 = call "数据处理整合 (子VI).vi"("枚举"=enum16{"实时数据排序", "小时数据排序"}."实时数据排序") -> ("已排序的数组"=w382:string[])  [unwired: 10 in]
            n344 = Array Size(array=w382) -> (size(s)=w381:i32)
            n345 = global write "全局 数据数组大小.vi" "数据数组大小"(w381) -> ()
          }
          frame #4 {
            # "判定是否存表"
            n346 = global read "全局 数据发送重叠.vi" "掉线指示灯"() -> (w383:bool)
            n347 = case shown="假" w383 {
              frame False {
                n348 = global read "全局 数据数组大小.vi" "数据数组大小"() -> (w384:i32)
                n349 = Greater Than 0?(x=w384) -> (x > 0?=w385:bool)
                n350 = case shown="真" w385 {
                  frame False {
                  }
                  frame True {
                    n351 = while {
                      stop <- w388 stop-if-true
                      n352 = global write "全局1.vi" "核查数据上传"(TRUE ("数据上传")) -> ()
                      n353 = Get Date/Time In Seconds() -> (seconds since 1Jan1904=w400:timestamp)
                      n354 = Format Date/Time String(time format string (%c)="%Y%m%d%H%M%S%3u" ("时间格式字符串(%c)"), seconds (now)=w400) -> (date/time string=w399:string)  [unwired: 1 in]
                      n355 = Search and Replace String(input string=w399, search string="." ("搜索字符串")) -> (result string=w397:string)  [unwired: 6 in, 3 out]
                      n356 = global read "断电保存全局.vi" "MN"() -> (w394:string)
                      n357 = global read "断电保存全局.vi" "PW"() -> (w393:string)
                      n358 = call "数据编码.vi"("table输入"="操作日志" ("新元素/子数组"), "QN"=w397, "MN"=w394, "PW"=w393) -> ("错误常量"=w392:errorcluster, "通讯包字符串"=w396:string)  [unwired: 10 in]
                      n359 = global read "全局 小时数据发送次数.vi" "小时数据发送次数"() -> (w389:i32)
                      n360 = global read "全局 数据数组大小.vi" "数据数组大小"() -> (w390:i32)
                      n361 = call "通信状态入队列.vi"("错误输入（无错误）"=w392, "枚举"=enum16{"打开连接", "发送数据", "读取数据", "数据处理", "关闭连接"}."发送数据") -> ()  [unwired: 9 in, 1 out]
                      n362 = global write "全局1.vi" "发送报文显示"(w396) -> ()
                      n363 = Decrement(x=w390) -> (x-1=w391:i32)
                      n364 = Greater Or Equal?(x=w389, y=w391) -> (x >= y?=w388:bool)
                      n365 = Wait (ms)(milliseconds to wait=u32 500 ("等待时间（毫秒）")) -> ()  [unwired: 1 out]
                    }
                  }
                }
              }
              frame True {
              }
            }
          }
        }
      }
      frame "仪器参数" {
        # "间隔时间上传"
        # "直接1分钟查询 一次,有数据就按数据上传,没数据就不上传,在数据发送那边有做处理"
        n366 = flat-sequence {
          frame #0 {
            n367 = global write "全局 小时数据发送次数.vi" "小时数据发送次数"(0 ("小时数据发送次数")) -> ()
            n368 = global write "全局1.vi" "枚举"(enum16{"返回请求应答", "上传数据", "返回执行结果"}."上传数据" ("枚举")) -> ()
          }
          frame #1 {
            n369 = call "获取操作日志 (子VI).vi"("table输入"="仪器参数") -> ()  [unwired: 11 in]
          }
          frame #2 {
            n370 = for {
              N: 5 -> [_]
              i -> [w409]
              # "行数大于零"
              n371 = case shown="3" w409 {
                tunnel: [w413 w414 w415 w416 w417] -> w408
                frame 0, Default {
                  n372 = global read "全局 所有参数.vi" "氨氮"() -> (w413:string[][])
                }
                frame 1 {
                  n373 = global read "全局 所有参数.vi" "总氮"() -> (w414:string[][])
                }
                frame 2 {
                  n374 = global read "全局 所有参数.vi" "总磷"() -> (w415:string[][])
                }
                frame 3 {
                  n375 = global read "全局 所有参数.vi" "CODMn"() -> (w416:string[][])
                }
                frame 4 {
                  n376 = global read "全局 所有参数.vi" "CODCr"() -> (w417:string[][])
                }
              }
              n377 = Array Size(array=w408) -> (size(s)=w411:i32[])
              n378 = Index Array(array=w411) -> (element=w410:i32)  [unwired: 1 in]
              n379 = Greater Than 0?(x=w410) -> (x > 0?=w412:bool)
              n380 = case shown="真" w412 {
                tunnel: w409 -> [_ w425]
                tunnel: w410 -> [_ _]
                tunnel: w408 -> [_ w420]
                frame False {
                }
                frame True {
                  # "最新时间戳加1分钟"
                  n381 = Array Size(array=w420) -> (size(s)=w422:i32[])
                  n382 = Index Array(array=w422) -> (element=w421:i32)  [unwired: 1 in]
                  n383 = Decrement(x=w421) -> (x-1=w419:i32)
                  n384 = Index Array(array=w420, index (row)=w419, index (col)=0 ("禁用的索引 (列)")) -> (element=w424:string)
                  n385 = call "日期时间字符串转换分钟数加一.vi"("data[0]"=w424) -> ("日期/时间字符串"=w423:string)  [unwired: 10 in]
                  n386 = case shown="3" w425 {
                    tunnel: w423 -> [w426 w427 w428 w429 w430]
                    frame 0, Default {
                      n387 = global write "全局 时间2.vi" "氨氮仪器参数索引起始时间"(w426) -> ()
                    }
                    frame 1 {
                      n388 = global write "全局 时间2.vi" "总氮仪器参数索引起始时间"(w427) -> ()
                    }
                    frame 2 {
                      n389 = global write "全局 时间2.vi" "总磷仪器参数索引起始时间"(w428) -> ()
                    }
                    frame 3 {
                      n390 = global write "全局 时间2.vi" "CODMn仪器参数索引起始时间"(w429) -> ()
                    }
                    frame 4 {
                      n391 = global write "全局 时间2.vi" "CODCr仪器参数索引起始时间"(w430) -> ()
                    }
                  }
                }
              }
            }
          }
          frame #3 {
            n392 = call "数据处理整合 (子VI).vi"("枚举"=enum16{"实时数据排序", "小时数据排序"}."实时数据排序") -> ("已排序的数组"=w433:string[])  [unwired: 10 in]
            n393 = Array Size(array=w433) -> (size(s)=w432:i32)
            n394 = global write "全局 数据数组大小.vi" "数据数组大小"(w432) -> ()
          }
          frame #4 {
            # "判定是否存表"
            n395 = global read "全局 数据发送重叠.vi" "掉线指示灯"() -> (w434:bool)
            n396 = case shown="假" w434 {
              frame False {
                n397 = global read "全局 数据数组大小.vi" "数据数组大小"() -> (w435:i32)
                n398 = Greater Than 0?(x=w435) -> (x > 0?=w436:bool)
                n399 = case shown="真" w436 {
                  frame False {
                  }
                  frame True {
                    n400 = while {
                      stop <- w438 stop-if-true
                      n401 = global write "全局1.vi" "核查数据上传"(TRUE ("数据上传")) -> ()
                      n402 = Get Date/Time In Seconds() -> (seconds since 1Jan1904=w451:timestamp)
                      n403 = Format Date/Time String(time format string (%c)="%Y%m%d%H%M%S%3u" ("时间格式字符串(%c)"), seconds (now)=w451) -> (date/time string=w450:string)  [unwired: 1 in]
                      n404 = Search and Replace String(input string=w450, search string="." ("搜索字符串")) -> (result string=w448:string)  [unwired: 6 in, 3 out]
                      n405 = global read "断电保存全局.vi" "MN"() -> (w445:string)
                      n406 = global read "断电保存全局.vi" "PW"() -> (w444:string)
                      n407 = global read "全局 数据数组大小.vi" "数据数组大小"() -> (w440:i32)
                      n408 = call "数据编码.vi"("table输入"="仪器参数" ("新元素/子数组"), "QN"=w448, "MN"=w445, "PW"=w444) -> ("错误常量"=w443:errorcluster, "通讯包字符串"=w447:string)  [unwired: 10 in]
                      n409 = global read "全局 小时数据发送次数.vi" "小时数据发送次数"() -> (w441:i32)
                      n410 = global write "全局1.vi" "发送报文显示"(w447) -> ()
                      n411 = call "通信状态入队列.vi"("错误输入（无错误）"=w443, "枚举"=enum16{"打开连接", "发送数据", "读取数据", "数据处理", "关闭连接"}."发送数据") -> ()  [unwired: 9 in, 1 out]
                      n412 = Decrement(x=w440) -> (x-1=w439:i32)
                      n413 = Greater Or Equal?(x=w441, y=w439) -> (x >= y?=w438:bool)
                      n414 = Wait (ms)(milliseconds to wait=u32 500 ("等待时间（毫秒）")) -> ()  [unwired: 1 out]
                    }
                  }
                }
              }
              frame True {
              }
            }
          }
        }
      }
      frame "系统状态" {
        # "直接1分钟查询 一次,有变化就按上传,没变化就不上传"
        n415 = flat-sequence {
          frame #0 {
            # "时间"
            n416 = global write "全局 小时数据发送次数.vi" "小时数据发送次数"(0 ("小时数据发送次数")) -> ()
            n417 = global write "全局 数据数组大小.vi" "数据数组大小"(1 ("数据数组大小")) -> ()
            n418 = global write "全局1.vi" "枚举"(enum16{"返回请求应答", "上传数据", "返回执行结果"}."上传数据" ("枚举")) -> ()
          }
          frame #1 {
            # "判定是否存表"
            n419 = global read "全局 数据发送重叠.vi" "掉线指示灯"() -> (w458:bool)
            n420 = case shown="假" w458 {
              frame False {
                n421 = global read "全局1.vi" "系统状态"() -> (w459:bool)
                n422 = case shown="真" w459 {
                  frame False {
                  }
                  frame True {
                    n423 = global read "全局 小时数据发送次数.vi" "小时数据发送次数"() -> (w468:i32)
                    n424 = global write "全局1.vi" "核查数据上传"(TRUE ("数据上传")) -> ()
                    n425 = global write "全局1.vi" "系统状态"(FALSE ("系统状态")) -> ()
                    n426 = Get Date/Time In Seconds() -> (seconds since 1Jan1904=w472:timestamp)
                    n427 = Increment(x=w468) -> (x+1=w467:i32)
                    n428 = Format Date/Time String(time format string (%c)="%Y%m%d%H%M%S%3u" ("时间格式字符串(%c)"), seconds (now)=w472) -> (date/time string=w471:string)  [unwired: 1 in]
                    n429 = global write "全局 小时数据发送次数.vi" "小时数据发送次数"(w467) -> ()
                    n430 = Search and Replace String(input string=w471, search string="." ("搜索字符串")) -> (result string=w469:string)  [unwired: 6 in, 3 out]
                    n431 = global read "断电保存全局.vi" "MN"() -> (w464:string)
                    n432 = global read "断电保存全局.vi" "PW"() -> (w463:string)
                    n433 = call "数据编码.vi"("table输入"="系统状态" ("新元素/子数组"), "QN"=w469, "MN"=w464, "PW"=w463) -> ("错误常量"=w462:errorcluster, "通讯包字符串"=w466:string)  [unwired: 10 in]
                    n434 = call "通信状态入队列.vi"("错误输入（无错误）"=w462, "枚举"=enum16{"打开连接", "发送数据", "读取数据", "数据处理", "关闭连接"}."发送数据") -> ()  [unwired: 9 in, 1 out]
                    n435 = global write "全局1.vi" "发送报文显示"(w466) -> ()
                  }
                }
              }
              frame True {
              }
            }
          }
        }
      }
      frame "运行模式" {
        # "直接1分钟查询 一次,有变化就按上传,没变化就不上传"
        n436 = flat-sequence {
          frame #0 {
            # "时间"
            n437 = global write "全局 小时数据发送次数.vi" "小时数据发送次数"(0 ("小时数据发送次数")) -> ()
            n438 = global write "全局 数据数组大小.vi" "数据数组大小"(1 ("数据数组大小")) -> ()
            n439 = global write "全局1.vi" "枚举"(enum16{"返回请求应答", "上传数据", "返回执行结果"}."上传数据" ("枚举")) -> ()
          }
          frame #1 {
            # "判定是否存表"
            n440 = global read "全局 数据发送重叠.vi" "掉线指示灯"() -> (w479:bool)
            n441 = case shown="假" w479 {
              frame False {
                n442 = global read "全局1.vi" "运行模式"() -> (w480:bool)
                n443 = case shown="真" w480 {
                  frame False {
                  }
                  frame True {
                    n444 = global read "全局 小时数据发送次数.vi" "小时数据发送次数"() -> (w489:i32)
                    n445 = global write "全局1.vi" "核查数据上传"(TRUE ("数据上传")) -> ()
                    n446 = global write "全局1.vi" "运行模式"(FALSE ("系统状态")) -> ()
                    n447 = Get Date/Time In Seconds() -> (seconds since 1Jan1904=w493:timestamp)
                    n448 = Increment(x=w489) -> (x+1=w488:i32)
                    n449 = Format Date/Time String(time format string (%c)="%Y%m%d%H%M%S%3u" ("时间格式字符串(%c)"), seconds (now)=w493) -> (date/time string=w492:string)  [unwired: 1 in]
                    n450 = global write "全局 小时数据发送次数.vi" "小时数据发送次数"(w488) -> ()
                    n451 = Search and Replace String(input string=w492, search string="." ("搜索字符串")) -> (result string=w490:string)  [unwired: 6 in, 3 out]
                    n452 = global read "断电保存全局.vi" "MN"() -> (w485:string)
                    n453 = global read "断电保存全局.vi" "PW"() -> (w484:string)
                    n454 = call "数据编码.vi"("table输入"="运行模式" ("新元素/子数组"), "QN"=w490, "MN"=w485, "PW"=w484) -> ("错误常量"=w483:errorcluster, "通讯包字符串"=w487:string)  [unwired: 10 in]
                    n455 = call "通信状态入队列.vi"("错误输入（无错误）"=w483, "枚举"=enum16{"打开连接", "发送数据", "读取数据", "数据处理", "关闭连接"}."发送数据") -> ()  [unwired: 9 in, 1 out]
                    n456 = global write "全局1.vi" "发送报文显示"(w487) -> ()
                  }
                }
              }
              frame True {
              }
            }
          }
        }
      }
      frame "测量周期" {
        # "直接1分钟查询 一次,有变化就按上传,没变化就不上传"
        n457 = flat-sequence {
          frame #0 {
            # "时间"
            n458 = global write "全局 小时数据发送次数.vi" "小时数据发送次数"(0 ("小时数据发送次数")) -> ()
            n459 = global write "全局 数据数组大小.vi" "数据数组大小"(1 ("数据数组大小")) -> ()
            n460 = global write "全局1.vi" "枚举"(enum16{"返回请求应答", "上传数据", "返回执行结果"}."上传数据" ("枚举")) -> ()
          }
          frame #1 {
            # "判定是否存表"
            n461 = global read "全局 数据发送重叠.vi" "掉线指示灯"() -> (w500:bool)
            n462 = case shown="假" w500 {
              frame False {
                n463 = global read "全局1.vi" "测量周期"() -> (w501:bool)
                n464 = case shown="真" w501 {
                  frame False {
                  }
                  frame True {
                    n465 = global read "全局 小时数据发送次数.vi" "小时数据发送次数"() -> (w510:i32)
                    n466 = global write "全局1.vi" "核查数据上传"(TRUE ("数据上传")) -> ()
                    n467 = global write "全局1.vi" "测量周期"(FALSE ("系统状态")) -> ()
                    n468 = Get Date/Time In Seconds() -> (seconds since 1Jan1904=w514:timestamp)
                    n469 = Increment(x=w510) -> (x+1=w509:i32)
                    n470 = Format Date/Time String(time format string (%c)="%Y%m%d%H%M%S%3u" ("时间格式字符串(%c)"), seconds (now)=w514) -> (date/time string=w513:string)  [unwired: 1 in]
                    n471 = global write "全局 小时数据发送次数.vi" "小时数据发送次数"(w509) -> ()
                    n472 = Search and Replace String(input string=w513, search string="." ("搜索字符串")) -> (result string=w511:string)  [unwired: 6 in, 3 out]
                    n473 = global read "断电保存全局.vi" "MN"() -> (w506:string)
                    n474 = global read "断电保存全局.vi" "PW"() -> (w505:string)
                    n475 = call "数据编码.vi"("table输入"="测量周期" ("新元素/子数组"), "QN"=w511, "MN"=w506, "PW"=w505) -> ("错误常量"=w504:errorcluster, "通讯包字符串"=w508:string)  [unwired: 10 in]
                    n476 = global write "全局1.vi" "发送报文显示"(w508) -> ()
                    n477 = call "通信状态入队列.vi"("错误输入（无错误）"=w504, "枚举"=enum16{"打开连接", "发送数据", "读取数据", "数据处理", "关闭连接"}."发送数据") -> ()  [unwired: 9 in, 1 out]
                  }
                }
              }
              frame True {
              }
            }
          }
        }
      }
      frame "超标留样" {
        # "直接1分钟查询 一次,有变化就按上传,没变化就不上传"
        n478 = flat-sequence {
          frame #0 {
            # "时间"
            n479 = global write "全局 小时数据发送次数.vi" "小时数据发送次数"(0 ("小时数据发送次数")) -> ()
            n480 = global write "全局 数据数组大小.vi" "数据数组大小"(1 ("数据数组大小")) -> ()
            n481 = global write "全局1.vi" "枚举"(enum16{"返回请求应答", "上传数据", "返回执行结果"}."上传数据" ("枚举")) -> ()
          }
          frame #1 {
            # "判定是否存表"
            n482 = global read "全局 数据发送重叠.vi" "掉线指示灯"() -> (w521:bool)
            n483 = case shown="假" w521 {
              frame False {
                n484 = global read "全局1.vi" "超标留样"() -> (w522:bool)
                n485 = case shown="真" w522 {
                  frame False {
                  }
                  frame True {
                    n486 = global read "全局 小时数据发送次数.vi" "小时数据发送次数"() -> (w531:i32)
                    n487 = global write "全局1.vi" "核查数据上传"(TRUE ("数据上传")) -> ()
                    n488 = global write "全局1.vi" "超标留样"(FALSE ("系统状态")) -> ()
                    n489 = Get Date/Time In Seconds() -> (seconds since 1Jan1904=w535:timestamp)
                    n490 = Increment(x=w531) -> (x+1=w530:i32)
                    n491 = Format Date/Time String(time format string (%c)="%Y%m%d%H%M%S%3u" ("时间格式字符串(%c)"), seconds (now)=w535) -> (date/time string=w534:string)  [unwired: 1 in]
                    n492 = global write "全局 小时数据发送次数.vi" "小时数据发送次数"(w530) -> ()
                    n493 = Search and Replace String(input string=w534, search string="." ("搜索字符串")) -> (result string=w532:string)  [unwired: 6 in, 3 out]
                    n494 = global read "断电保存全局.vi" "MN"() -> (w526:string)
                    n495 = global read "断电保存全局.vi" "PW"() -> (w525:string)
                    n496 = call "数据编码.vi"("table输入"="超标留样" ("新元素/子数组"), "QN"=w532, "MN"=w526, "PW"=w525) -> ("错误常量"=w527:errorcluster, "通讯包字符串"=w529:string)  [unwired: 10 in]
                    n497 = global write "全局1.vi" "发送报文显示"(w529) -> ()
                    n498 = call "通信状态入队列.vi"("错误输入（无错误）"=w527, "枚举"=enum16{"打开连接", "发送数据", "读取数据", "数据处理", "关闭连接"}."发送数据") -> ()  [unwired: 9 in, 1 out]
                  }
                }
              }
              frame True {
              }
            }
          }
        }
      }
      frame "报警信息" {
        # "间隔时间上传"
        # "直接1分钟查询 一次,有数据就按数据上传,没数据为空的不传,在数据发送那边有做处理"
        n499 = flat-sequence {
          frame #0 {
            # "分钟时间间隔"
            n500 = call "日志信息主动发送(子VI).vi"() -> ()  [unwired: 12 in]
            n501 = global write "全局 小时数据发送次数.vi" "小时数据发送次数"(0 ("小时数据发送次数")) -> ()
            n502 = global write "全局1.vi" "枚举"(enum16{"返回请求应答", "上传数据", "返回执行结果"}."上传数据" ("枚举")) -> ()
          }
          frame #1 {
            n503 = call "获取报警信息 (子VI).vi"() -> ()  [unwired: 12 in]
          }
          frame #2 {
            n504 = for {
              N: 12 -> [_]
              i -> [w543]
              # "行数大于零"
              n505 = case shown="0, 默认" w543 {
                tunnel: [w547 w548 w549 w550 w551 w552 w553 w554 w555 w556 w557 w558] -> w542
                frame 0, Default {
                  n506 = global read "全局 所有参数.vi" "氨氮"() -> (w547:string[][])
                }
                frame 1 {
                  n507 = global read "全局 所有参数.vi" "总氮"() -> (w548:string[][])
                }
                frame 2 {
                  n508 = global read "全局 所有参数.vi" "总磷"() -> (w549:string[][])
                }
                frame 3 {
                  n509 = global read "全局 所有参数.vi" "CODMn"() -> (w550:string[][])
                }
                frame 4 {
                  n510 = global read "全局 所有参数.vi" "CODCr"() -> (w551:string[][])
                }
                frame 5 {
                  n511 = global read "全局 所有参数.vi" "DO"() -> (w552:string[][])
                }
                frame 6 {
                  n512 = global read "全局 所有参数.vi" "PH"() -> (w553:string[][])
                }
                frame 7 {
                  n513 = global read "全局 所有参数.vi" "电导率"() -> (w554:string[][])
                }
                frame 8 {
                  n514 = global read "全局 所有参数.vi" "水温"() -> (w555:string[][])
                }
                frame 9 {
                  n515 = global read "全局 所有参数.vi" "浊度"() -> (w556:string[][])
                }
                frame 10 {
                  n516 = global read "全局 所有参数.vi" "叶绿素"() -> (w557:string[][])
                }
                frame 11 {
                  n517 = global read "全局 所有参数.vi" "藻密度"() -> (w558:string[][])
                }
              }
              n518 = Array Size(array=w542) -> (size(s)=w545:i32[])
              n519 = Index Array(array=w545) -> (element=w544:i32)  [unwired: 1 in]
              n520 = Greater Than 0?(x=w544) -> (x > 0?=w546:bool)
              n521 = case shown="真" w546 {
                tunnel: w543 -> [_ w566]
                tunnel: w544 -> [_ _]
                tunnel: w542 -> [_ w561]
                frame False {
                }
                frame True {
                  # "最新时间戳加1分钟"
                  n522 = Array Size(array=w561) -> (size(s)=w563:i32[])
                  n523 = Index Array(array=w563) -> (element=w562:i32)  [unwired: 1 in]
                  n524 = Decrement(x=w562) -> (x-1=w560:i32)
                  n525 = Index Array(array=w561, index (row)=w560, index (col)=0 ("禁用的索引 (列)")) -> (element=w565:string)
                  n526 = call "日期时间字符串转换分钟数加一.vi"("data[0]"=w565) -> ("日期/时间字符串"=w564:string)  [unwired: 10 in]
                  n527 = case shown="0, 默认" w566 {
                    tunnel: w564 -> [w567 w568 w569 w570 w571 w572 w573 w574 w575 w576 w577 w578]
                    frame 0, Default {
                      n528 = global write "全局 时间2.vi" "氨氮报警信息索引起始时间"(w567) -> ()
                    }
                    frame 1 {
                      n529 = global write "全局 时间2.vi" "总氮报警信息索引起始时间"(w568) -> ()
                    }
                    frame 2 {
                      n530 = global write "全局 时间2.vi" "总磷报警信息索引起始时间"(w569) -> ()
                    }
                    frame 3 {
                      n531 = global write "全局 时间2.vi" "CODMn报警信息索引起始时间"(w570) -> ()
                    }
                    frame 4 {
                      n532 = global write "全局 时间2.vi" "CODCr报警信息索引起始时间"(w571) -> ()
                    }
                    frame 5 {
                      n533 = global write "全局 时间2.vi" "DO报警信息索引起始时间"(w572) -> ()
                    }
                    frame 6 {
                      n534 = global write "全局 时间2.vi" "PH报警信息索引起始时间"(w573) -> ()
                    }
                    frame 7 {
                      n535 = global write "全局 时间2.vi" "比电导率报警信息索引起始时间"(w574) -> ()
                    }
                    frame 8 {
                      n536 = global write "全局 时间2.vi" "水温报警信息索引起始时间"(w575) -> ()
                    }
                    frame 9 {
                      n537 = global write "全局 时间2.vi" "浊度报警信息索引起始时间"(w576) -> ()
                    }
                    frame 10 {
                      n538 = global write "全局 时间2.vi" "叶绿素报警信息索引起始时间"(w577) -> ()
                    }
                    frame 11 {
                      n539 = global write "全局 时间2.vi" "系统报警信息索引起始时间"(w578) -> ()
                    }
                  }
                }
              }
            }
          }
          frame #3 {
            n540 = call "数据处理整合 (子VI).vi"("枚举"=enum16{"实时数据排序", "小时数据排序"}."实时数据排序") -> ("已排序的数组"=w581:string[])  [unwired: 10 in]
            n541 = Array Size(array=w581) -> (size(s)=w580:i32)
            n542 = global write "全局 数据数组大小.vi" "数据数组大小"(w580) -> ()
          }
          frame #4 {
            # "判定是否存表"
            n543 = global read "全局 数据发送重叠.vi" "掉线指示灯"() -> (w582:bool)
            n544 = case shown="假" w582 {
              frame False {
                # "判定数据不为空才发"
                n545 = global read "全局 数据数组大小.vi" "数据数组大小"() -> (w583:i32)
                n546 = Greater Than 0?(x=w583) -> (x > 0?=w584:bool)
                n547 = case shown="真" w584 {
                  frame False {
                    n548 = global write "全局1.vi" "核查数据上传"(FALSE ("数据上传")) -> ()
                  }
                  frame True {
                    n549 = while {
                      stop <- w587 stop-if-true
                      n550 = Wait (ms)(milliseconds to wait=u32 500 ("等待时间（毫秒）")) -> ()  [unwired: 1 out]
                      n551 = Get Date/Time In Seconds() -> (seconds since 1Jan1904=w599:timestamp)
                      n552 = Format Date/Time String(time format string (%c)="%Y%m%d%H%M%S%3u" ("时间格式字符串(%c)"), seconds (now)=w599) -> (date/time string=w598:string)  [unwired: 1 in]
                      n553 = global read "全局 数据数组大小.vi" "数据数组大小"() -> (w589:i32)
                      n554 = Search and Replace String(input string=w598, search string="." ("搜索字符串")) -> (result string=w596:string)  [unwired: 6 in, 3 out]
                      n555 = global read "断电保存全局.vi" "MN"() -> (w593:string)
                      n556 = global read "断电保存全局.vi" "PW"() -> (w592:string)
                      n557 = global read "全局 小时数据发送次数.vi" "小时数据发送次数"() -> (w590:i32)
                      n558 = call "数据编码.vi"("table输入"="报警信息" ("新元素/子数组"), "QN"=w596, "MN"=w593, "PW"=w592) -> ("错误常量"=w591:errorcluster, "通讯包字符串"=w595:string)  [unwired: 10 in]
                      n559 = Decrement(x=w589) -> (x-1=w588:i32)
                      n560 = global write "全局1.vi" "发送报文显示"(w595) -> ()
                      n561 = Greater Or Equal?(x=w590, y=w588) -> (x >= y?=w587:bool)
                      n562 = call "通信状态入队列.vi"("错误输入（无错误）"=w591, "枚举"=enum16{"打开连接", "发送数据", "读取数据", "数据处理", "关闭连接"}."发送数据") -> ()  [unwired: 9 in, 1 out]
                    }
                  }
                }
              }
              frame True {
              }
            }
          }
        }
      }
      frame "环境参数" {
      }
    }
  }
  "错误输出" <- w1
